vi "posterior estimate covariance.vi"(10 "Pk|k-1":T1, 11 "K_k":T1) -> (3 "Pk|k":T1)   [LabVIEW 2016]
uses:
  <vilib>/Analysis/Matrix/Datatypes/RealMatrix.ctl
  <vilib>/Analysis/Matrix/Numeric/Multiply/Multiply - RM,RM.vi
  <vilib>/Analysis/Matrix/Numeric/Subtract/Subtract - RM,RM.vi
  <vilib>/Analysis/Matrix/NI_Matrix.lvlib
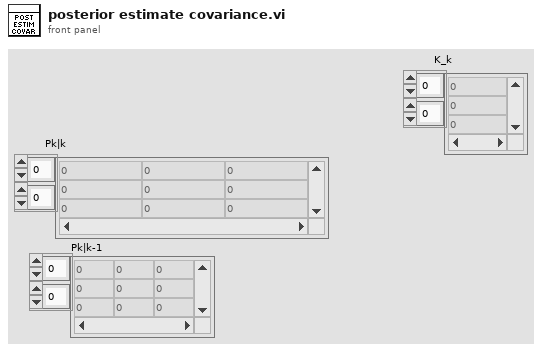
[diagram p1: front panel]
types:
  T1 = typedef "NI_Matrix.lvlib/RealMatrix.ctl" = dbl[][]
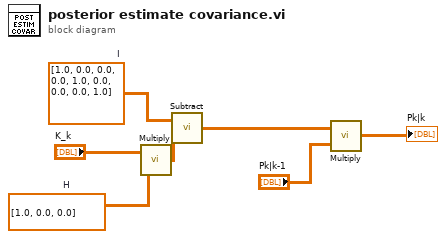
[diagram p0: block diagram]
diagram:
  w3 = T1 [[1.0, 0.0, 0.0]]  # H
  w6 = T1 [[1.0, 0.0, 0.0], [0.0, 1.0, 0.0], [0.0, 0.0, 1.0]]  # I
  n1 = call-poly <vilib>:"Multiply.vi"("Real Matrix B"=w3, "Real Matrix A"="K_k") -> ("A * B"=w7:T1)
  n2 = call-poly <vilib>:"Subtract.vi"("Real Matrix B"=w7, "Real Matrix A"=w6) -> ("A - B"=w5:T1)
  n3 = call-poly <vilib>:"Multiply.vi"("Real Matrix B"="Pk|k-1", "Real Matrix A"=w5) -> ("A * B"=→"Pk|k":T1)
